vi "Ramp.vi"(4 "i":i32=10001, 6 "phase":dbl, 7 "function (ramp)":enum16{"Ramp", "Triangle", "Sine"}(ring), 8 "cycles (1,2,...)":i32=1 min=1 step=1, 9 "step size":dbl=0.001 format="%.4f", 10 "offset":dbl=5.0 format="%0.2f", 11 "amplitude":dbl=5.0 format="%0.2f") -> (0 "stop?":bool=TRUE, 2 "Waveform Graph":dbl[](graph), 3 "element":dbl)   [LabVIEW 2016]
uses:
  <vilib>/Analysis/1siggen.llb/Ramp Pattern by Delta.vi
  <vilib>/Analysis/NI_AALBase.lvlib
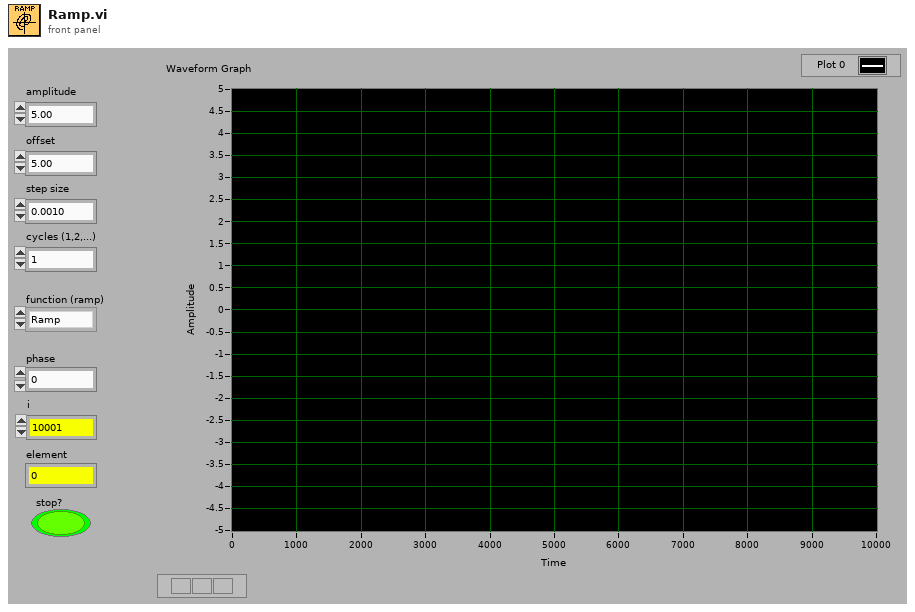
[diagram p1: front panel]
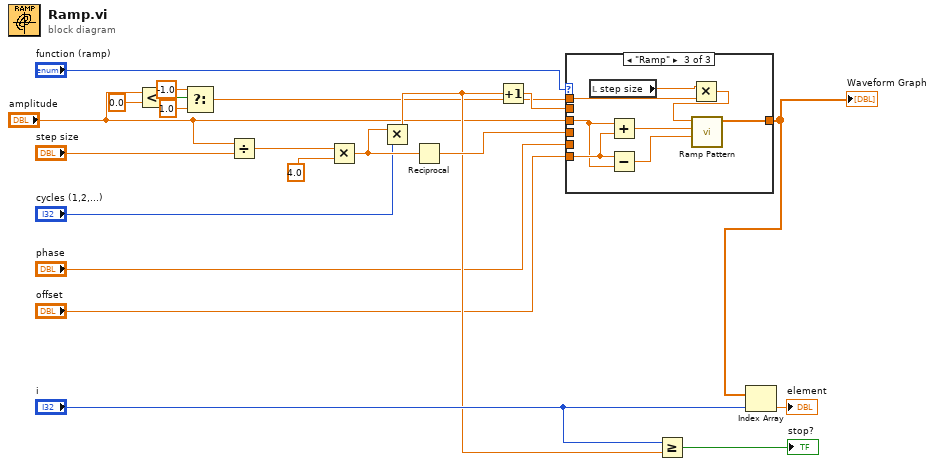
[diagram p0: block diagram]
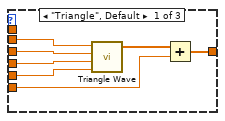
[diagram p2: hidden frame]
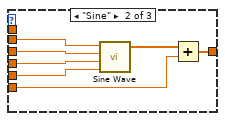
[diagram p3: hidden frame]
diagram:
  n1 = Less?(x="amplitude", y=0.0) -> (x < y?=w4:bool)
  n2 = Select(t=-1.0, s=w4, f=1.0) -> (s? t:f=w1:dbl)
  n3 = Divide(x="amplitude", y="step size") -> (x/y=w21:dbl)
  n4 = Multiply(x=w21, y=4.0) -> (x*y=w14:dbl)
  n5 = Multiply(x=w14, y="cycles (1,2,...)") -> (x*y=w13:dbl)
  n6 = Reciprocal(x=w14) -> (1/x=w15:dbl)
  n7 = Increment(x=w13) -> (x+1=w17:dbl)
  n8 = case shown="\"Ramp\"" "function (ramp)" {
    tunnel: "amplitude" -> [w28 w34 w41]
    tunnel: [w24 w31 w43] -> w10
    tunnel: w15 -> [w27 w33 _]
    tunnel: w17 -> [w26 w35 _]
    tunnel: "phase" -> [w25 w32 _]
    tunnel: "offset" -> [w22 w29 w42]
    tunnel: w1 -> [_ _ w38]
    frame "Triangle", Default {
      n9 = call <vilib>:"Triangle Wave.vi"("samples"=w26, "amplitude"=w28, "frequency"=w27, "phase in"=w25) -> ("triangle wave"=w23:dbl[])  [unwired: 1 in, 2 out]
      n10 = Add(x=w23, y=w22) -> (x+y=w24:dbl[])
    }
    frame "Sine" {
      n11 = call <vilib>:"Sine Wave.vi"("samples"=w35, "amplitude"=w34, "frequency"=w33, "phase in"=w32) -> ("sine wave"=w30:dbl[])  [unwired: 1 in, 2 out]
      n12 = Add(x=w30, y=w29) -> (x+y=w31:dbl[])
    }
    frame "Ramp" {
      n13 = local read "step size"() -> (w37:dbl)
      n14 = Add(x=w41, y=w42) -> (x+y=w39:dbl)
      n15 = Subtract(x=w42, y=w41) -> (x-y=w40:dbl)
      n16 = Multiply(x=w37, y=w38) -> (x*y=w36:dbl)
      n17 = call-poly <vilib>:"Ramp Pattern.vi"("start"=w40, "end"=w39, "delta"=w36) -> ("Ramp Pattern"=w43:dbl[])  [unwired: 6 in, 2 out]
    }
  }
  "Waveform Graph" <- w10
  n18 = Greater Or Equal?(x="i", y=w13) -> (x >= y?=→"stop?":bool)
  n19 = Index Array(array=w10, index="i") -> (element=→"element":dbl)
